vi "check_sum.vi"(11 "command":string) -> (3 "Check Sum":string)   [LabVIEW 2015]
panel:
  out "byte":u8
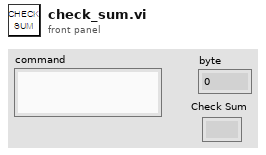
[diagram p1: front panel]
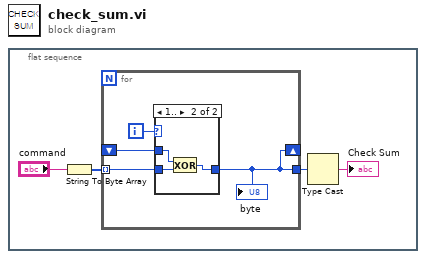
[diagram p0: block diagram]
diagram:
  n1 = flat-sequence {
    frame #0 {
      n2 = String To Byte Array(string="command") -> (unsigned byte array=w4:u8[])
      n3 = for {
        shift-right: [w5] -> _
        shift-left: _ -> [w6]
        tunnel: w4 -> [w7] mode=indexing
        tunnel: [w5] -> w1
        i -> [w8]
        n4 = case shown="1.." w8 {
          tunnel: [w9 w10] -> w5
          tunnel: w7 -> [w9 w11]
          tunnel: w6 -> [_ w12]
          frame 0, Default {
          }
          frame 1.. {
            n5 = Exclusive Or(1:w11, 2:w12) -> (0:w10:u8)
          }
        }
        "byte" <- w5
      }
      n6 = Type Cast(x=w1) -> (*(type *) &x=→"Check Sum":string)  [unwired: 1 in]
    }
  }
